vi "Broadcast Response.vi"(6 "Controller name":string, 8 "error in (no error)":errorcluster, 9 "Update period":dbl, 11 "Measure Object in":refnum<class "Simple Sequencer.lvclass">) -> (0 "error out":errorcluster, 3 "Measure Object out":refnum<class "Simple Sequencer.lvclass">)   [LabVIEW 2024, in "Simple Sequencer.lvclass"]
uses:
  Simple Sequencer.lvclass
  Simple Sequencer.lvclass/Simple Sequencer.ctl
  NHMFL_Core/Libraries/Instruments/Results/Acquired Result/Acquired Result.lvclass
panel:
  in  "Topic":string
  in  "Acquired Result.lvclass":refnum<class "Acquired Result.lvclass">
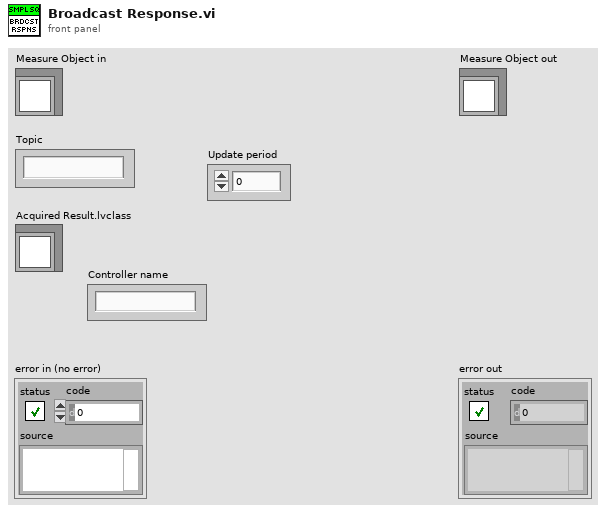
[diagram p1: front panel]
types:
  T1 = typedef "Simple Sequencer Configuration.ctl" = cluster{"Primary instrument":string, "Secondary instrument":string, "Start":dbl, "End":dbl, "Step":dbl, "Secondary start":dbl, "Secondary end":dbl}
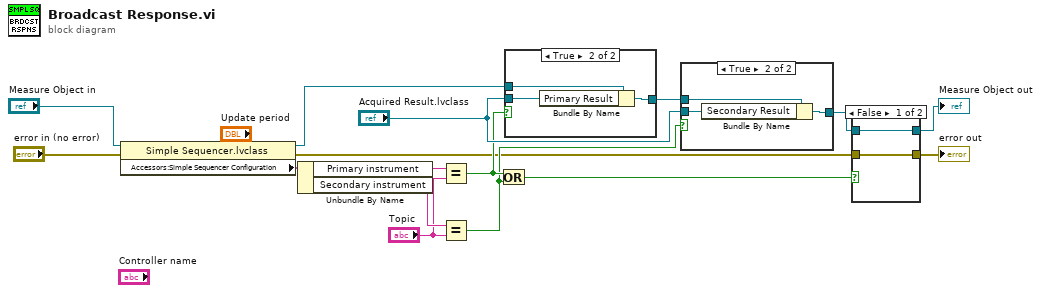
[diagram p0: block diagram]
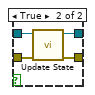
[diagram p2: hidden frame]
diagram:
  n1 = property class="Simple Sequencer.lvclass"(reference="Measure Object in", error in="error in (no error)") -> (reference out=w11:refnum<class "Simple Sequencer.lvclass">, error out=w2:errorcluster, "Accessors:Simple Sequencer Configuration"=w16:T1)
  n2 = Unbundle By Name(w16) -> ("Primary instrument"=w13:string, "Secondary instrument"=w15:string)
  n3 = Equal?(x=w13, y="Topic") -> (x = y?=w8:bool)
  n4 = Equal?(x=w15, y="Topic") -> (x = y?=w7:bool)
  n5 = Or(x=w8, y=w7) -> (x .or. y?=w1:bool)
  n6 = case shown="True" w8 {
    tunnel: w11 -> [w17 w20]
    tunnel: "Acquired Result.lvclass" -> [_ w19]
    tunnel: [w17 w18] -> w10
    frame False {
    }
    frame True {
      n7 = Bundle By Name(cluster=w20, "Primary Result"=w19) -> (w18:refnum<class "Simple Sequencer.lvclass">)
    }
  }
  n8 = case shown="True" w7 {
    tunnel: w10 -> [w21 w24]
    tunnel: "Acquired Result.lvclass" -> [_ w23]
    tunnel: [w21 w22] -> w6
    frame False {
    }
    frame True {
      n9 = Bundle By Name(cluster=w24, "Secondary Result"=w23) -> (w22:refnum<class "Simple Sequencer.lvclass">)
    }
  }
  n10 = case shown="False" w1 {
    tunnel: w6 -> [w26 w30]
    tunnel: w2 -> [w25 w29]
    tunnel: [w25 w28] -> w5
    tunnel: [w26 w27] -> w4
    frame False {
    }
    frame True {
      n11 = call-dynamic "Update State.vi"("error in (no error)"=w29, "Simple Sequencer in"=w30) -> ("error out"=w28:errorcluster, "Simple Sequencer out"=w27:refnum<class "Simple Sequencer.lvclass">)  [unwired: 8 in]
    }
  }
  "error out" <- w5
  "Measure Object out" <- w4
